vi "LCR_TrimOC.vi"(8 "error in (no error)":errorcluster, 11 "LCRControl in":refnum<class "LCRControl.lvclass">) -> (0 "error out":errorcluster, 3 "LCRControl out":refnum<class "LCRControl.lvclass">)   [LabVIEW 2018, in "LCRControl.lvclass"]
uses:
  LCRControl.lvclass
  C:/Users/itkstriplabview4/Documents/itk-strip-sensor-qc/InstrControl/InstrControl.lvclass
  InstrControl.lvclass
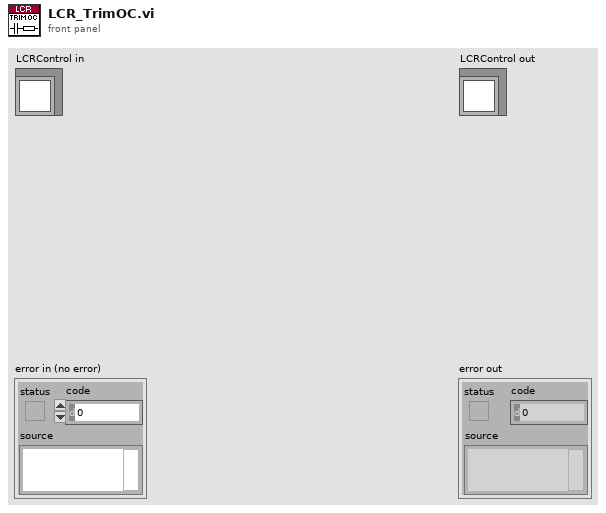
[diagram p1: front panel]
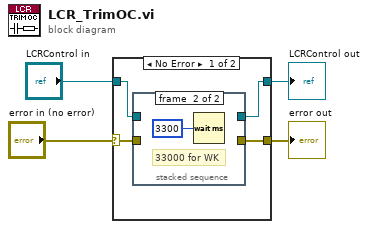
[diagram p0: block diagram]
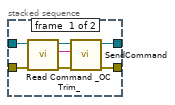
[diagram p2: hidden frame]
diagram:
  n1 = case shown="No Error" "error in (no error)" {
    selector: "error in (no error)" -> [w5 w18]
    tunnel: [w7 w18] -> w3
    tunnel: [w8 w17] -> w1
    tunnel: "LCRControl in" -> [w6 w17]
    frame No Error {
      n2 = stacked-sequence {
        tunnel: [w15 _] -> w8
        tunnel: w5 -> [w11 _]
        tunnel: [w10 _] -> w7
        tunnel: w6 -> [w9 _]
        frame #0 {
          n3 = call-dynamic "Read Command _OC Trim_.vi"("error in (no error)"=w11, "LCRControl in"=w9) -> ("error out"=w12:errorcluster, "Command \"OC Trim\""=w13:string, "LCRControl out"=w14:refnum<class "LCRControl.lvclass">)  [unwired: 7 in]
          n4 = call "SendCommand.vi"("error in (no error)"=w12, "Command string"=w13, "InstControl in"=w14) -> ("error out"=w10:errorcluster, "InstControl out"=w15:refnum<class "LCRControl.lvclass">)  [unwired: 7 in]
        }
        frame #1 {
          # "33000 for WK"
          n5 = Wait (ms)(milliseconds to wait=3300) -> ()  [unwired: 1 out]
        }
      }
    }
    frame Error {
    }
  }
  "error out" <- w3
  "LCRControl out" <- w1
